vi "SetupMove.vi"(8 "error in (no error)":errorcluster, 10 "moveDestination":dbl, 11 "KST101 in":refnum<class "KST101.lvclass">) -> (0 "error out":errorcluster, 3 "KST101 out":refnum<class "KST101.lvclass">)   [LabVIEW 2016, in "Stepper Motor Controller.lvlib" / "KST101.lvclass"]
uses:
  KST101.lvclass
  KST101.lvclass/KST101.ctl
  D:/Workspace/ProCyteOne_LaserModuleAlignment/shared/Thorlabs/Kinesis/Dependencies/Thorlabs.MotionControl.KCube.StepperMotorCLI.dll
  Dependencies/Thorlabs.MotionControl.KCube.StepperMotorCLI.dll
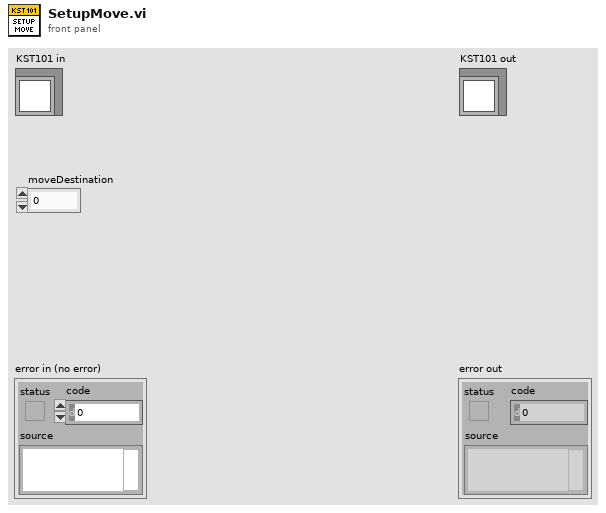
[diagram p1: front panel]
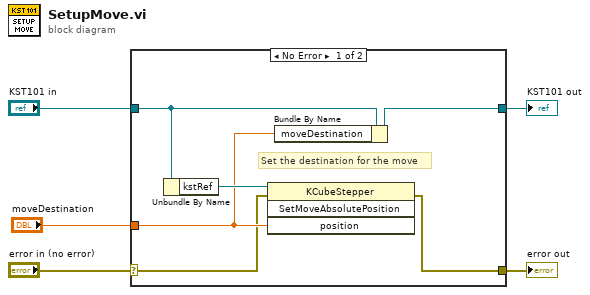
[diagram p0: block diagram]
diagram:
  n1 = case shown="No Error" "error in (no error)" {
    selector: "error in (no error)" -> [w7 w13]
    tunnel: [w6 w13] -> w4
    tunnel: [w9 w12] -> w2
    tunnel: "KST101 in" -> [w10 w12]
    tunnel: "moveDestination" -> [w8 _]
    frame No Error {
      # "Set the destination for the move"
      n2 = Unbundle By Name(w10) -> ("kstRef"=w11:refnum<k24>)
      n3 = invoke class="KCubeStepper" method="SetMoveAbsolutePosition"(reference=w11, error in=w7, "position"=w8) -> (error out=w6:errorcluster)  [unwired: 1 in, 3 out]
      n4 = Bundle By Name(cluster=w10, "moveDestination"=w8) -> (w9:refnum<class "KST101.lvclass">)
    }
    frame Error {
    }
  }
  "error out" <- w4
  "KST101 out" <- w2
